vi "Update Stack.vi"(7 "Device":refnum<class "Device.lvclass">, 8 "error in (no error)":errorcluster, 11 "Stack in":refnum<class "Device.lvclass">[](array[class])) -> (0 "error out":errorcluster, 3 "Stack out":refnum<class "Device.lvclass">[](array[class]))   [LabVIEW 2011, in "Tinkerforge.lvlib" / "Device.lvclass"]
doc: "This VI updates the stack and inserts the <B>Device</B> into the <B>Stack</B>."
uses:
  Device.lvclass
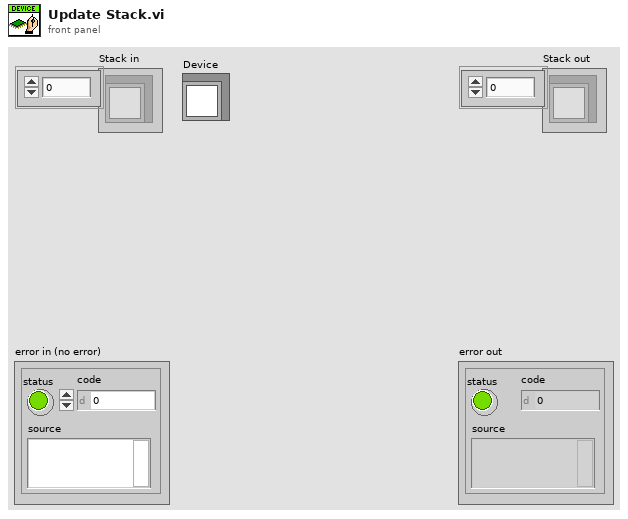
[diagram p1: front panel]
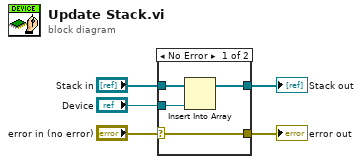
[diagram p0: block diagram]
diagram:
  n1 = case shown="No Error" "error in (no error)" {
    selector: "error in (no error)" -> [w8 w11]
    tunnel: [w8 w11] -> w4
    tunnel: [w9 w10] -> w2
    tunnel: "Stack in" -> [w7 w10]
    tunnel: "Device" -> [w6 _]
    frame No Error {
      n2 = Insert Into Array(array=w7, new element=w6) -> (w9:refnum<class "Device.lvclass">[])  [unwired: 1 in]
    }
    frame Error {
    }
  }
  "error out" <- w4
  "Stack out" <- w2
